vi "czyGotoweDoPomiaru.vi"() -> (3 "Czy gotowe?":bool)   [LabVIEW 2014]
uses:
  parametryKomorVIs/WyborKomory.ctl
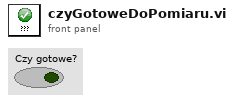
[diagram p1: front panel]
types:
  T1 = typedef "WyborKomory.ctl" = enum16{"NADAWCZA", "ODBIORCZA"}
  T2 = typedef "Gotowosc.ctl" = cluster{"Poziomy":bool, "Pionowy":bool}
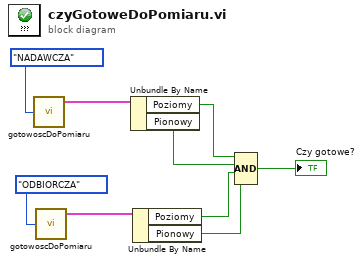
[diagram p0: block diagram]
diagram:
  n1 = call "gotowoscDoPomiaru.vi"("Wybór komory"=WyborKomory."NADAWCZA") -> ("Gotowoœæ wyjœcie"=w1:T2)  [unwired: 4 in]
  n2 = call "gotowoscDoPomiaru.vi"("Wybór komory"=WyborKomory."ODBIORCZA") -> ("Gotowoœæ wyjœcie"=w2:T2)  [unwired: 4 in]
  n3 = Unbundle By Name(w1) -> ("Poziomy"=w4:bool, "Pionowy"=w5:bool)
  n4 = Unbundle By Name(w2) -> ("Poziomy"=w6:bool, "Pionowy"=w7:bool)
  n5 = Compound Arithmetic op=AND(w4, w5, w6, w7) -> (→"Czy gotowe?":bool)
